vi "TLB Native Dynamic Events ver 0.01.vi"() -> ()   [LabVIEW 2018]
uses:
  Labview Training Phase 2/Enum Controls/States for Action Engine.ctl
  <vilib>/myRIO/Instrument Drivers/Onboard IO/DIO/typedefs/DIO Reference.ctl
  <vilib>/myRIO/Common/Instrument Driver Framework/Utilities/typedefs/myRIO Generic Hardware Reference.ctl
  <vilib>/myRIO/Common/Instrument Driver Framework/Utilities/typedefs/Hardware Version Enum.ctl
  <vilib>/myRIO/Common/Instrument Driver Framework/Utilities/typedefs/myRIO v1.0 Reference.ctl
  <vilib>/myRIO/Common/Instrument Driver Framework/Utilities/typedefs/Generic FPGA Reference.ctl
  <vilib>/myRIO/Common/Instrument Driver Framework/myRIO v1.0/DIO/typedefs/DIO Channels List.ctl
  <vilib>/myRIO/Common/Instrument Driver Framework/myRIO v1.0/DIO/typedefs/DIO Channels Enum.ctl
  <vilib>/userdefined/High Color/nirio_resource_hc.ctl
  <vilib>/myRIO/Common/Instrument Driver Framework/Utilities/vis/Is FPGA Ref Available.vi
  <vilib>/myRIO/Common/Instrument Driver Framework/myRIO v1.0/DIO/vis/myRIO v1.1 Open DIO.vi
  <vilib>/myRIO/Instrument Drivers/Onboard IO/DIO/vis/Write.vi
  <vilib>/myRIO/Common/Instrument Driver Framework/Utilities/vis/Validate Channels.vi
  <vilib>/myRIO/Common/Instrument Driver Framework/myRIO v1.0/DIO/vis/myRIO v1.0 Reserve DIO.vi
  <vilib>/myRIO/Common/Instrument Driver Framework/myRIO v1.0/Resource Manager/vis/myRIO v1.0 Reserve Channel List.vi
  <vilib>/myRIO/Common/Instrument Driver Framework/myRIO v1.0/DIO/vis/myRIO v1.0 Build MUX Configuration DIO.vi
  <vilib>/myRIO/Common/Instrument Driver Framework/myRIO v1.0/Resource Manager/vis/myRIO v1.0 Reserve Channel.vi
  <vilib>/myRIO/Common/Instrument Driver Framework/myRIO v1.0/Resource Manager/vis/myRIO v1.0 Unreserve Channel.vi
  <vilib>/myRIO/Common/Instrument Driver Framework/myRIO v1.0/Resource Manager/vis/myRIO v1.0 Create Configuration List.vi
  <vilib>/myRIO/Common/Instrument Driver Framework/myRIO v1.0/Resource Manager/vis/myRIO v1.0 Build Mutex Name.vi
  <vilib>/Utility/VariantDataType/GetNumericInfo.vi
  <vilib>/Utility/error.llb/Error Cluster From Error Code.vi
  <vilib>/myRIO/Common/Instrument Driver Framework/myRIO v1.0/myRIO v1.1 Open.vi
  <vilib>/myRIO/Common/Instrument Driver Framework/Utilities/vis/IO Manager.vi
  <vilib>/myRIO/Common/Instrument Driver Framework/Utilities/vis/Configuration Manager.vi
  <vilib>/myRIO/Common/Instrument Driver Framework/myRIO v1.0/Resource Manager/vis/myRIO v1.0 Configure IO.vi
  <vilib>/myRIO/Common/Instrument Driver Framework/myRIO v1.0/myRIO v1.0 Close.vi
  <vilib>/myRIO/Common/Instrument Driver Framework/myRIO v1.0/DIO/vis/myRIO v1.0 Write DIO.vi
  <vilib>/myRIO/Express VI/Onboard Devices/LED/LED Express VI.xnode
  <vilib>/myRIO/Instrument Drivers/Onboard IO/DIO/vis/myRIO DIO Open.xnode
  <vilib>/myRIO/Instrument Drivers/Onboard IO/DIO/DIO.lvlib
panel:
  in  "Stop Queue":bool
  in  "Start Queue":bool
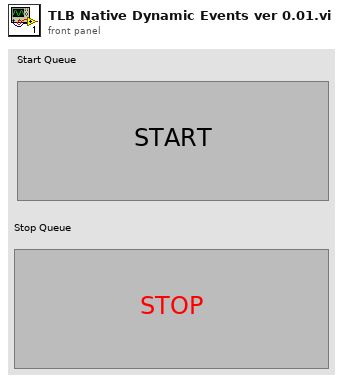
[diagram p1: front panel]
types:
  T1 = typedef "States for Action Engine.ctl" = enum16{"Initialize", "Write", "Read"}
  T2 = typedef "DIO.lvlib/DIO Reference.ctl" = cluster{"myRIO Reference":T3, "DIO Channels List":T7}
  T3 = typedef "myRIO Generic Hardware Reference.ctl" = cluster{"myRIO Model":T4, "myRIO Hardware Reference":T5}
  T4 = typedef "Hardware Version Enum.ctl" = enum16{"Unknown", "myRIO-1900", "myRIO-1950", "roboRIO", "NI ELVIS RIO CM", "ELVIS III"}
  T5 = typedef "myRIO v1.0 Reference.ctl" = cluster{"Generic FPGA Reference":T6, "Allow multiple opens":bool}
  T6 = typedef "Generic FPGA Reference.ctl" = refnum<k20>
  T7 = typedef "DIO Channels List.ctl" = T8[]
  T8 = typedef "DIO Channels Enum.ctl" = enum16{"Not Connected", "C/DIO0", "C/DIO1", "C/DIO2", "C/DIO3", "C/DIO4", "C/DIO5", "C/DIO6", "C/DIO7", "A/DIO0", "A/DIO1", "A/DIO2", "A/DIO3", "A/DIO4", "A/DIO5", "A/DIO6", "A/DIO7", "A/DIO8", "A/DIO9", "A/DIO10", "A/DIO11", "A/DIO12", "A/DIO13", "A/DIO14", "A/DIO15", "A/DIO16", "A/DIO17", "A/DIO18", "A/DIO19", "B/DIO0", "B/DIO1", "B/DIO2", "B/DIO3", "B/DIO4", "B/DIO5", "B/DIO6", "B/DIO7", "B/DIO8", "B/DIO9", "B/DIO10", "B/DIO11", "B/DIO12", "B/DIO13", "B/DIO14", "B/DIO15", "B/DIO16", "B/DIO17", "B/DIO18", "B/DIO19", "LED0", "LED1", "LED2", "LED3", "Button0", "DIO/DIO0", "DIO/DIO1", "DIO/DIO2", "DIO/DIO3", "DIO/DIO4", "DIO/DIO5", "DIO/DIO6", "DIO/DIO7", "DIO/DIO8", "DIO/DIO9", "SPI/CS0", "SPI/CS1", "SPI/CS2", "SPI/CS3", "LED RADIO (Green)", "LED RADIO (Red)", "LED COMM (Green)", "LED COMM (Red)", "LED MODE (Green)", "LED MODE (Red)"}
  T9 = typedef "nirio_resource_hc.ctl" = tag
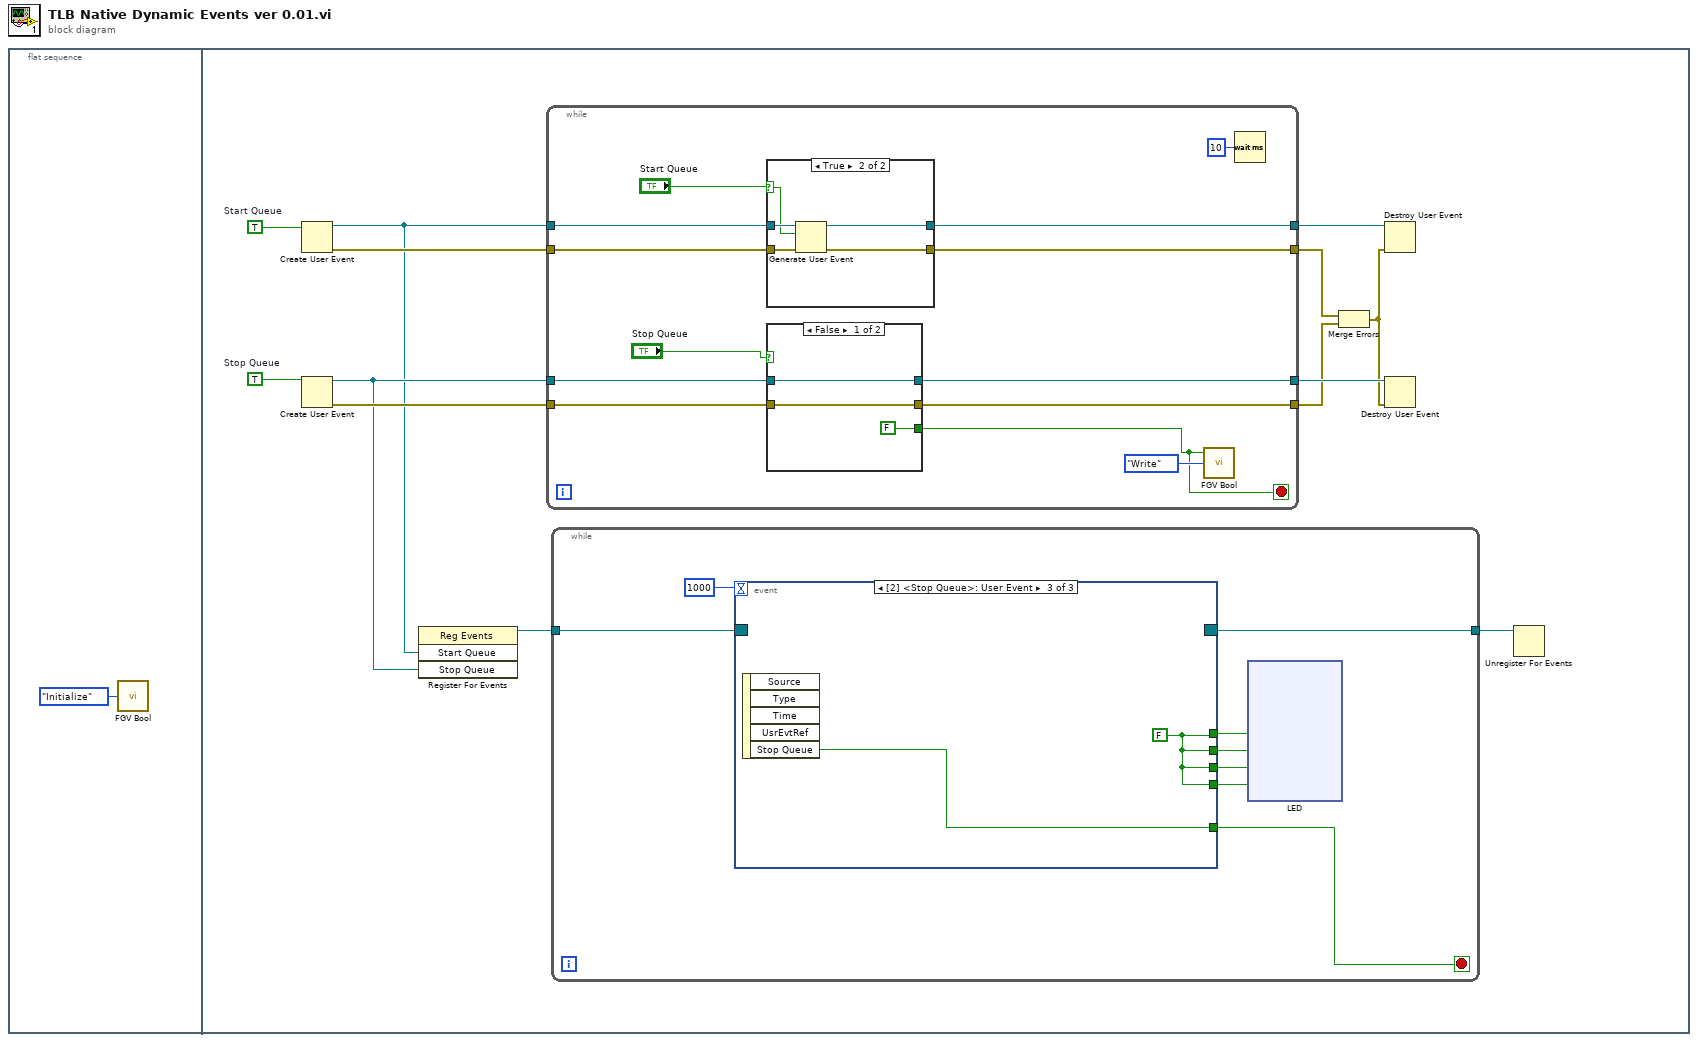
[diagram p0: block diagram]
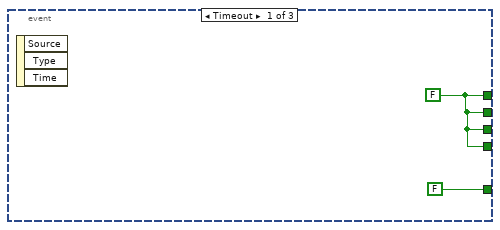
[diagram p2: hidden frame]
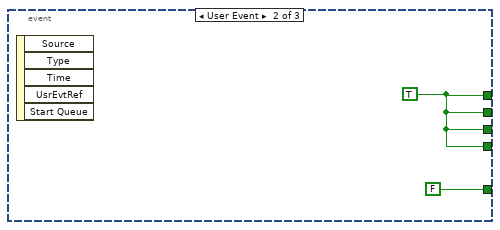
[diagram p3: hidden frame]
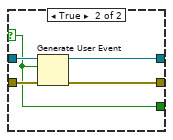
[diagram p4: hidden frame]
diagram:
  n1 = flat-sequence {
    frame #0 {
      n2 = call "FGV Bool.vi"("Init/Read/Write State"=States_for_Action_Engine."Initialize") -> ()  [unwired: 2 in, 2 out]
    }
    frame #1 {
      w14 = TRUE  # Stop Queue
      w13 = TRUE  # Start Queue
      n3 = Create User Event(user event datatype=w13) -> (user event=w4:refnum<user-event>, error out=w10:errorcluster)  [unwired: 1 in]
      n4 = Create User Event(user event datatype=w14) -> (user event=w5:refnum<user-event>, error out=w9:errorcluster)  [unwired: 1 in]
      n5 = register-events(w4, w5) -> (reference out=w3:refnum<event-registration>)  [unwired: 2 in, 1 out]
      n6 = while {
        tunnel: w4 -> [w78]
        tunnel: w5 -> [w77]
        tunnel: [w76] -> w12
        tunnel: [w75] -> w11
        tunnel: w10 -> [w74]
        tunnel: [w73] -> w8
        tunnel: w9 -> [w72]
        tunnel: [w71] -> w7
        stop <- w67 stop-if-true
        n7 = case shown="True" "Start Queue" {
          selector: "Start Queue" -> [_ w90]
          tunnel: w78 -> [w89 w94]
          tunnel: [w89 w93] -> w75
          tunnel: w74 -> [w88 w92]
          tunnel: [w88 w91] -> w73
          frame False {
          }
          frame True {
            n8 = Generate User Event(user event=w94, event data cluster=w90, error in=w92) -> (user event out=w93:refnum<user-event>, error out=w91:errorcluster)  [unwired: 1 in]
          }
        }
        n9 = case shown="False" "Stop Queue" {
          selector: "Stop Queue" -> [_ w83]
          tunnel: w77 -> [w82 w87]
          tunnel: [w82 w86] -> w76
          tunnel: w72 -> [w81 w85]
          tunnel: [w81 w84] -> w71
          tunnel: [FALSE w83] -> w67
          frame False {
          }
          frame True {
            n10 = Generate User Event(user event=w87, event data cluster=w83, error in=w85) -> (user event out=w86:refnum<user-event>, error out=w84:errorcluster)  [unwired: 1 in]
          }
        }
        n11 = call "FGV Bool.vi"("Init/Read/Write State"=States_for_Action_Engine."Write", "Input Node"=w67) -> ()  [unwired: 1 in, 2 out]
        n12 = Wait (ms)(milliseconds to wait=u32 10) -> ()  [unwired: 1 out]
      }
      n13 = while {
        tunnel: w3 -> [w21]
        tunnel: [w20] -> w2
        stop <- w15 stop-if-true
        n14 = event shown="[2] <Stop Queue>: User Event" {
          selector: w21 -> [_ _ _]
          dyn-events: [_ _ _] -> w20
          timeout: 1000 -> [_ _ _]
          tunnel: [w24 w26 w28] -> w19
          tunnel: [w24 w26 w28] -> w18
          tunnel: [w24 w26 w28] -> w17
          tunnel: [w24 w26 w28] -> w16
          tunnel: [FALSE FALSE w27] -> w15
          event Timeout {
            w24 = FALSE
            n15 = event-data() -> ()  [unwired: 1 in, 3 out]
          }
          event User Event {
            w26 = TRUE
            n16 = event-data() -> ()  [unwired: 1 in, 5 out]
          }
          event User Event {
            w28 = FALSE
            n17 = event-data() -> ("Stop Queue"=w27:bool)  [unwired: 1 in, 4 out]
          }
        }
        n18 = xnode "LED"("LED0"=w19, "LED1"=w18, "LED2"=w17, "LED3"=w16) -> ()  [unwired: 1 in, 1 out]
      }
      n19 = Merge Errors(w8, w7) -> (w6:errorcluster)
      n20 = Destroy User Event(user event=w11, error in=w6) -> ()  [unwired: 1 out]
      n21 = Destroy User Event(user event=w12, error in=w6) -> ()  [unwired: 1 out]
      n22 = Unregister For Events(event registration refnum=w2) -> ()  [unwired: 1 in, 1 out]
    }
  }
